vi "DeviceDestroy.vi"(7 "error in (no error)":errorcluster, 11 "Handle In":u64[](array[numeric])) -> (5 "error out":errorcluster)   [LabVIEW 2020, in "SnapMB.lvlib"]
uses:
  SnapMB.lvlib
  windows/snapmb.dll
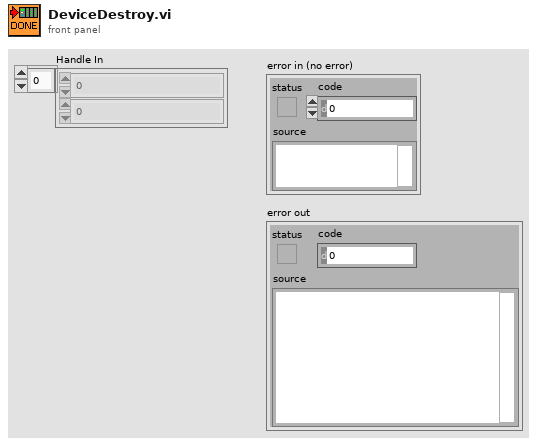
[diagram p1: front panel]
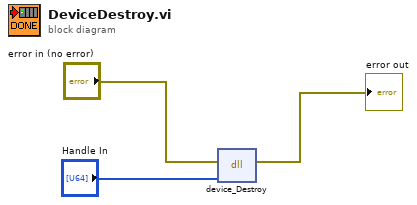
[diagram p0: block diagram]
diagram:
  n1 = dll-call lib="D:/SnapMB/LabView/lib/windows/snapmb.dll" fn="device_Destroy"(error in="error in (no error)", "Device"="Handle In") -> (error out=→"error out":errorcluster)  [unwired: 4 in, 1 out]
